vi "Event Log.vi"(8 "error in (no error)":errorcluster, 10 "Content":string, 11 "EVENT LOG":string) -> (0 "error out":errorcluster, 3 "EVENT LOG":string)   [LabVIEW 2025]
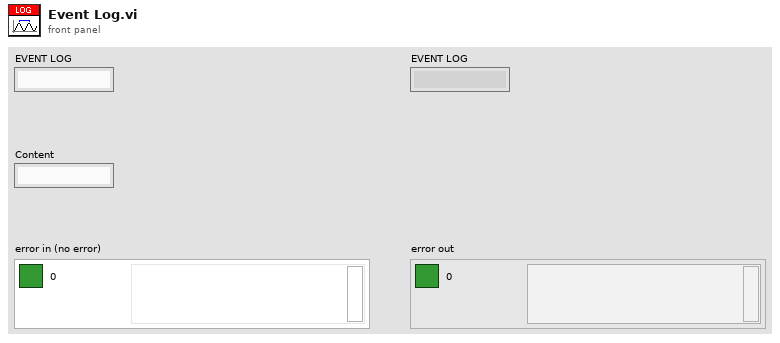
[diagram p1: front panel]
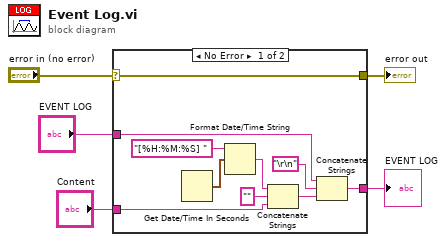
[diagram p0: block diagram]
diagram:
  n1 = case shown="No Error" "error in (no error)" {
    selector: "error in (no error)" -> [w6 _]
    tunnel: "EVENT LOG" -> [w9 _]
    tunnel: [w8 w16] -> w2
    tunnel: "Content" -> [w7 w16]
    tunnel: [w6 _] -> w5
    frame No Error {
      n2 = Get Date/Time In Seconds() -> (seconds since 1Jan1904=w12:timestamp)
      n3 = Format Date/Time String(time format string (%c)="[%H:%M:%S] ", seconds (now)=w12) -> (date/time string=w14:string)  [unwired: 1 in]
      n4 = Concatenate Strings(w14, "", w7) -> (w11:string)
      n5 = Concatenate Strings(w9, "\r\n", w11) -> (w8:string)
    }
    frame Error {
    }
  }
  "error out" <- w5
  "EVENT LOG" <- w2
